vi "Parameter Configuration.vi"(11 "当前项目选择":refnum<vi>) -> ()   [LabVIEW 2018]
uses:
  <vilib>/Utility/file.llb/Read From Spreadsheet File (string).vi
  <vilib>/Utility/file.llb/Write To Spreadsheet File (string).vi
panel:
  in  "手动信息输入":string[][](table)
  in  "确定按钮":bool
  in  "退出":bool
  # "项目设置"
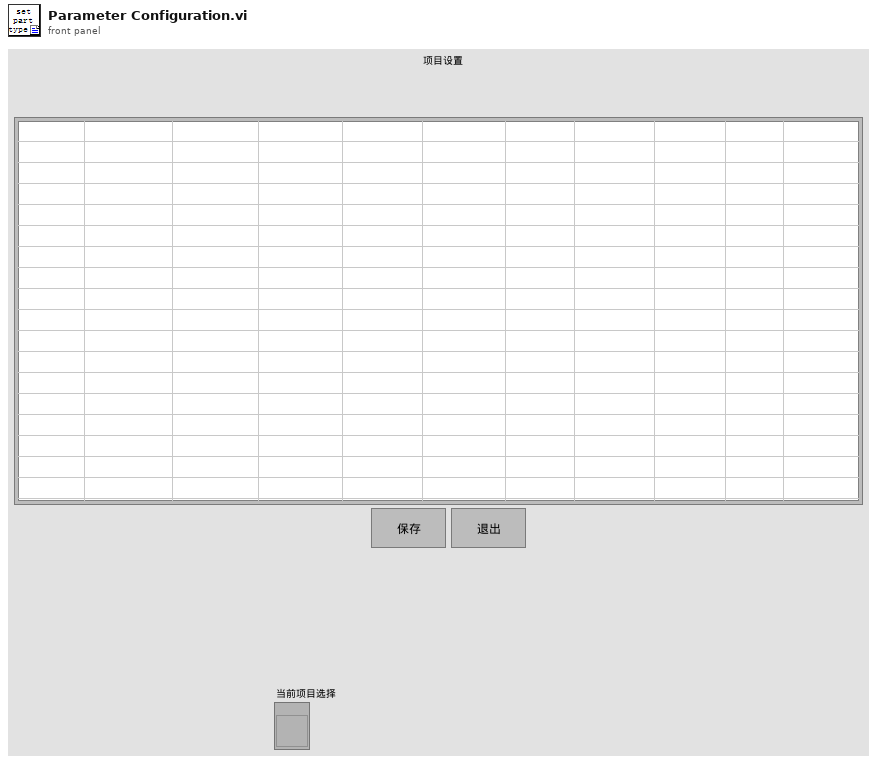
[diagram p1: front panel]
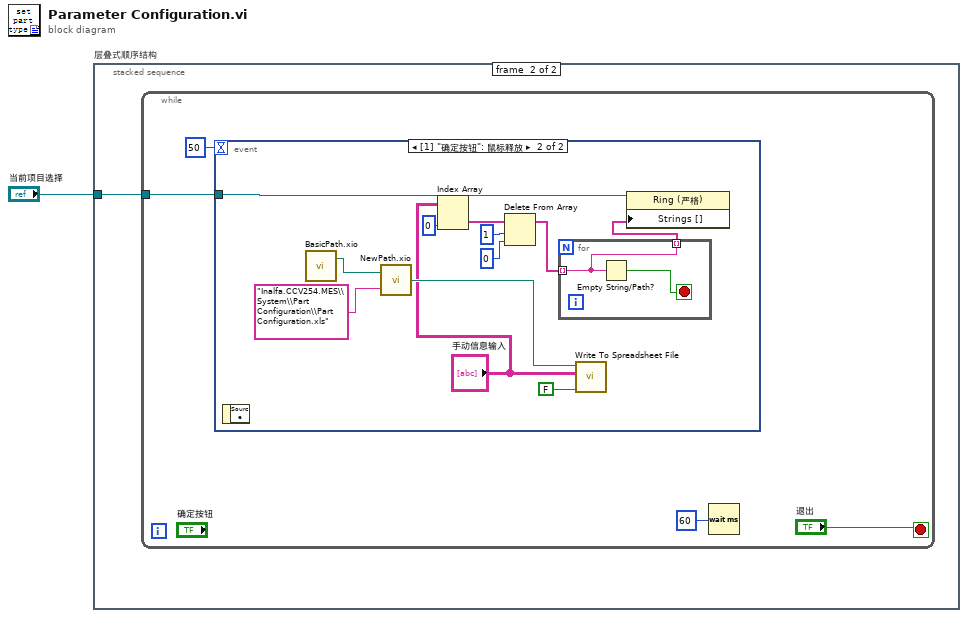
[diagram p0: block diagram]
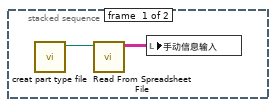
[diagram p2: hidden frame]
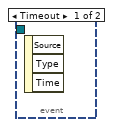
[diagram p3: hidden frame]
diagram:
  n1 = stacked-sequence "层叠式顺序结构" {
    tunnel: "当前项目选择" -> [_ w4]
    frame #0 {
      n2 = call "creat part type file.vi"() -> ("new file path (Not A Path if cancelled)"=w2:path)  [unwired: 11 in]
      n3 = call-poly <vilib>:"Read From Spreadsheet File.vi"("file path (dialog if empty)"=w2) -> ("all rows"=w3:string[][])  [unwired: 6 in, 4 out]
      n4 = local write "手动信息输入"(w3) -> ()
    }
    frame #1 {
      n5 = while {
        tunnel: w4 -> [w5]
        stop <- "退出" stop-if-true
        n6 = event shown="[1] \"确定按钮\": 鼠标释放" {
          selector: _ -> [_ _]
          dyn-events: _ -> [_ _]
          timeout: 50 -> [_ _]
          tunnel: w5 -> [_ w16]
          event Timeout {
            n7 = event-data() -> ()  [unwired: 1 in, 3 out]
          }
          event "确定按钮": Mouse Up {
            n8 = event-data() -> ()  [unwired: 1 in, 1 out]
            n9 = call "BasicPath.xio.vi"() -> ("stripped path"=w19:path)  [unwired: 1 in, 1 out]
            n10 = call "NewPath.xio.vi"("Append path"="Inalfa.CCV254.MES\\System\\Part Configuration\\Part Configuration.xls", "Basic path"=w19) -> ("New path"=w17:path)
            n11 = Index Array(array="手动信息输入", index (col)=0 ("禁用的索引 (列)")) -> (element=w13:string[])  [unwired: 1 in]
            n12 = Delete From Array(array=w13, length=1 ("长度"), index=0 ("索引")) -> (array with subset deleted=w10:string[])  [unwired: 1 out]
            n13 = for {
              tunnel: w10 -> [w21] mode=indexing
              tunnel: [w21] -> w9 mode=indexing
              stop <- w22 stop-if-true
              n14 = Empty String/Path?(string/path=w21) -> (empty?=w22:bool)
            }
            n15 = call-poly <vilib>:"Write To Spreadsheet File.vi"("append to file? (new file:F)"=FALSE, "2D data"="手动信息输入", "file path (dialog if empty)"=w17) -> ()  [unwired: 5 in, 1 out]
            n16 = property class="Ring (严格)"(reference=w16, "Strings []"=w9) -> ()  [unwired: 1 in, 2 out]
          }
        }
        n17 = Wait (ms)(milliseconds to wait=u32 60 ("等待时间（毫秒）")) -> ()  [unwired: 1 out]
      }
    }
  }
